vi "BoxExecute.vi"   [LabVIEW 2023]
uses:
  <vilib>/Rock Robotics/Network Tables/NT Write Number.vi
  <vilib>/Rock Robotics/Network Tables/NT Read Number.vi
  <vilib>/Rock Robotics/WPI/ThirdParty/JAS_Junk/TrajLib/Trajectory_Library.lvlib
  <vilib>/Rock Robotics/Network Tables/NT Write Boolean.vi
panel:
  # "Click here to set max"
  # "Click here to set min"
types:
  T1 = typedef "WPI_MotorControlDeviceRef.ctl" = cluster{"DeviceStatus":errorcluster, "Type":T2, "PWM":cluster{"PWM Channel":T3, "DeadBand":T4}, "CAN":cluster{"Device Number":u8, "SetOutput VI Ref":variant, "GetOutput VI Ref":variant, "Enable VI Ref":variant, "Disable VI Ref":variant, "Data":variant}, "Invert":bool, "DIO PWM":cluster{"PWM \"Enable\" Channel":T3, "DIOChannel":T5, "PWM Rate":dbl}}
  T2 = typedef "WPI_MotorControlType.ctl" = enum16{"PWM", "CAN", "DIO PWM"}
  T3 = typedef "FPGA_DIOPWMChannel.ctl" = enum8{"PWM 0", "PWM 1", "PWM 2", "PWM 3", "PWM 4", "PWM 5", "PWM 6", "PWM 7", "PWM 8", "PWM 9", "PWM MXP 0", "PWM MXP 1", "PWM MXP 2", "PWM MXP 3", "PWM MXP 4", "PWM MXP 5", "PWM MXP 6", "PWM MXP 7", "PWM MXP 8", "PWM MXP 9", "Invalid"}
  T4 = typedef "WPI_PWMDeadband.ctl" = cluster{"Name":string, "maxPositivePwm":i32, "minPositivePwm":i32, "centerPwm":i32, "maxNegativePwm":i32, "minNegativePwm":i32, "angularRange":u16}
  T5 = typedef "FPGA_DIOChannel.ctl" = enum8{"DIO 0", "DIO 1", "DIO 2", "DIO 3", "DIO 4", "DIO 5", "DIO 6", "DIO 7", "DIO 8", "DIO 9", "DIO MXP 0", "DIO MXP 1", "DIO MXP 2", "DIO MXP 3", "DIO MXP 4", "DIO MXP 5", "DIO MXP 6", "DIO MXP 7", "DIO MXP 8", "DIO MXP 9", "DIO MXP 10", "DIO MXP 11", "DIO MXP 12", "DIO MXP 13", "DIO MXP 14", "DIO MXP 15", "SPI Port CS1", "SPI Port CS2", "SPI Port CS3", "SPI Port MISO", "SPI Port MOSI", "Invalid"}
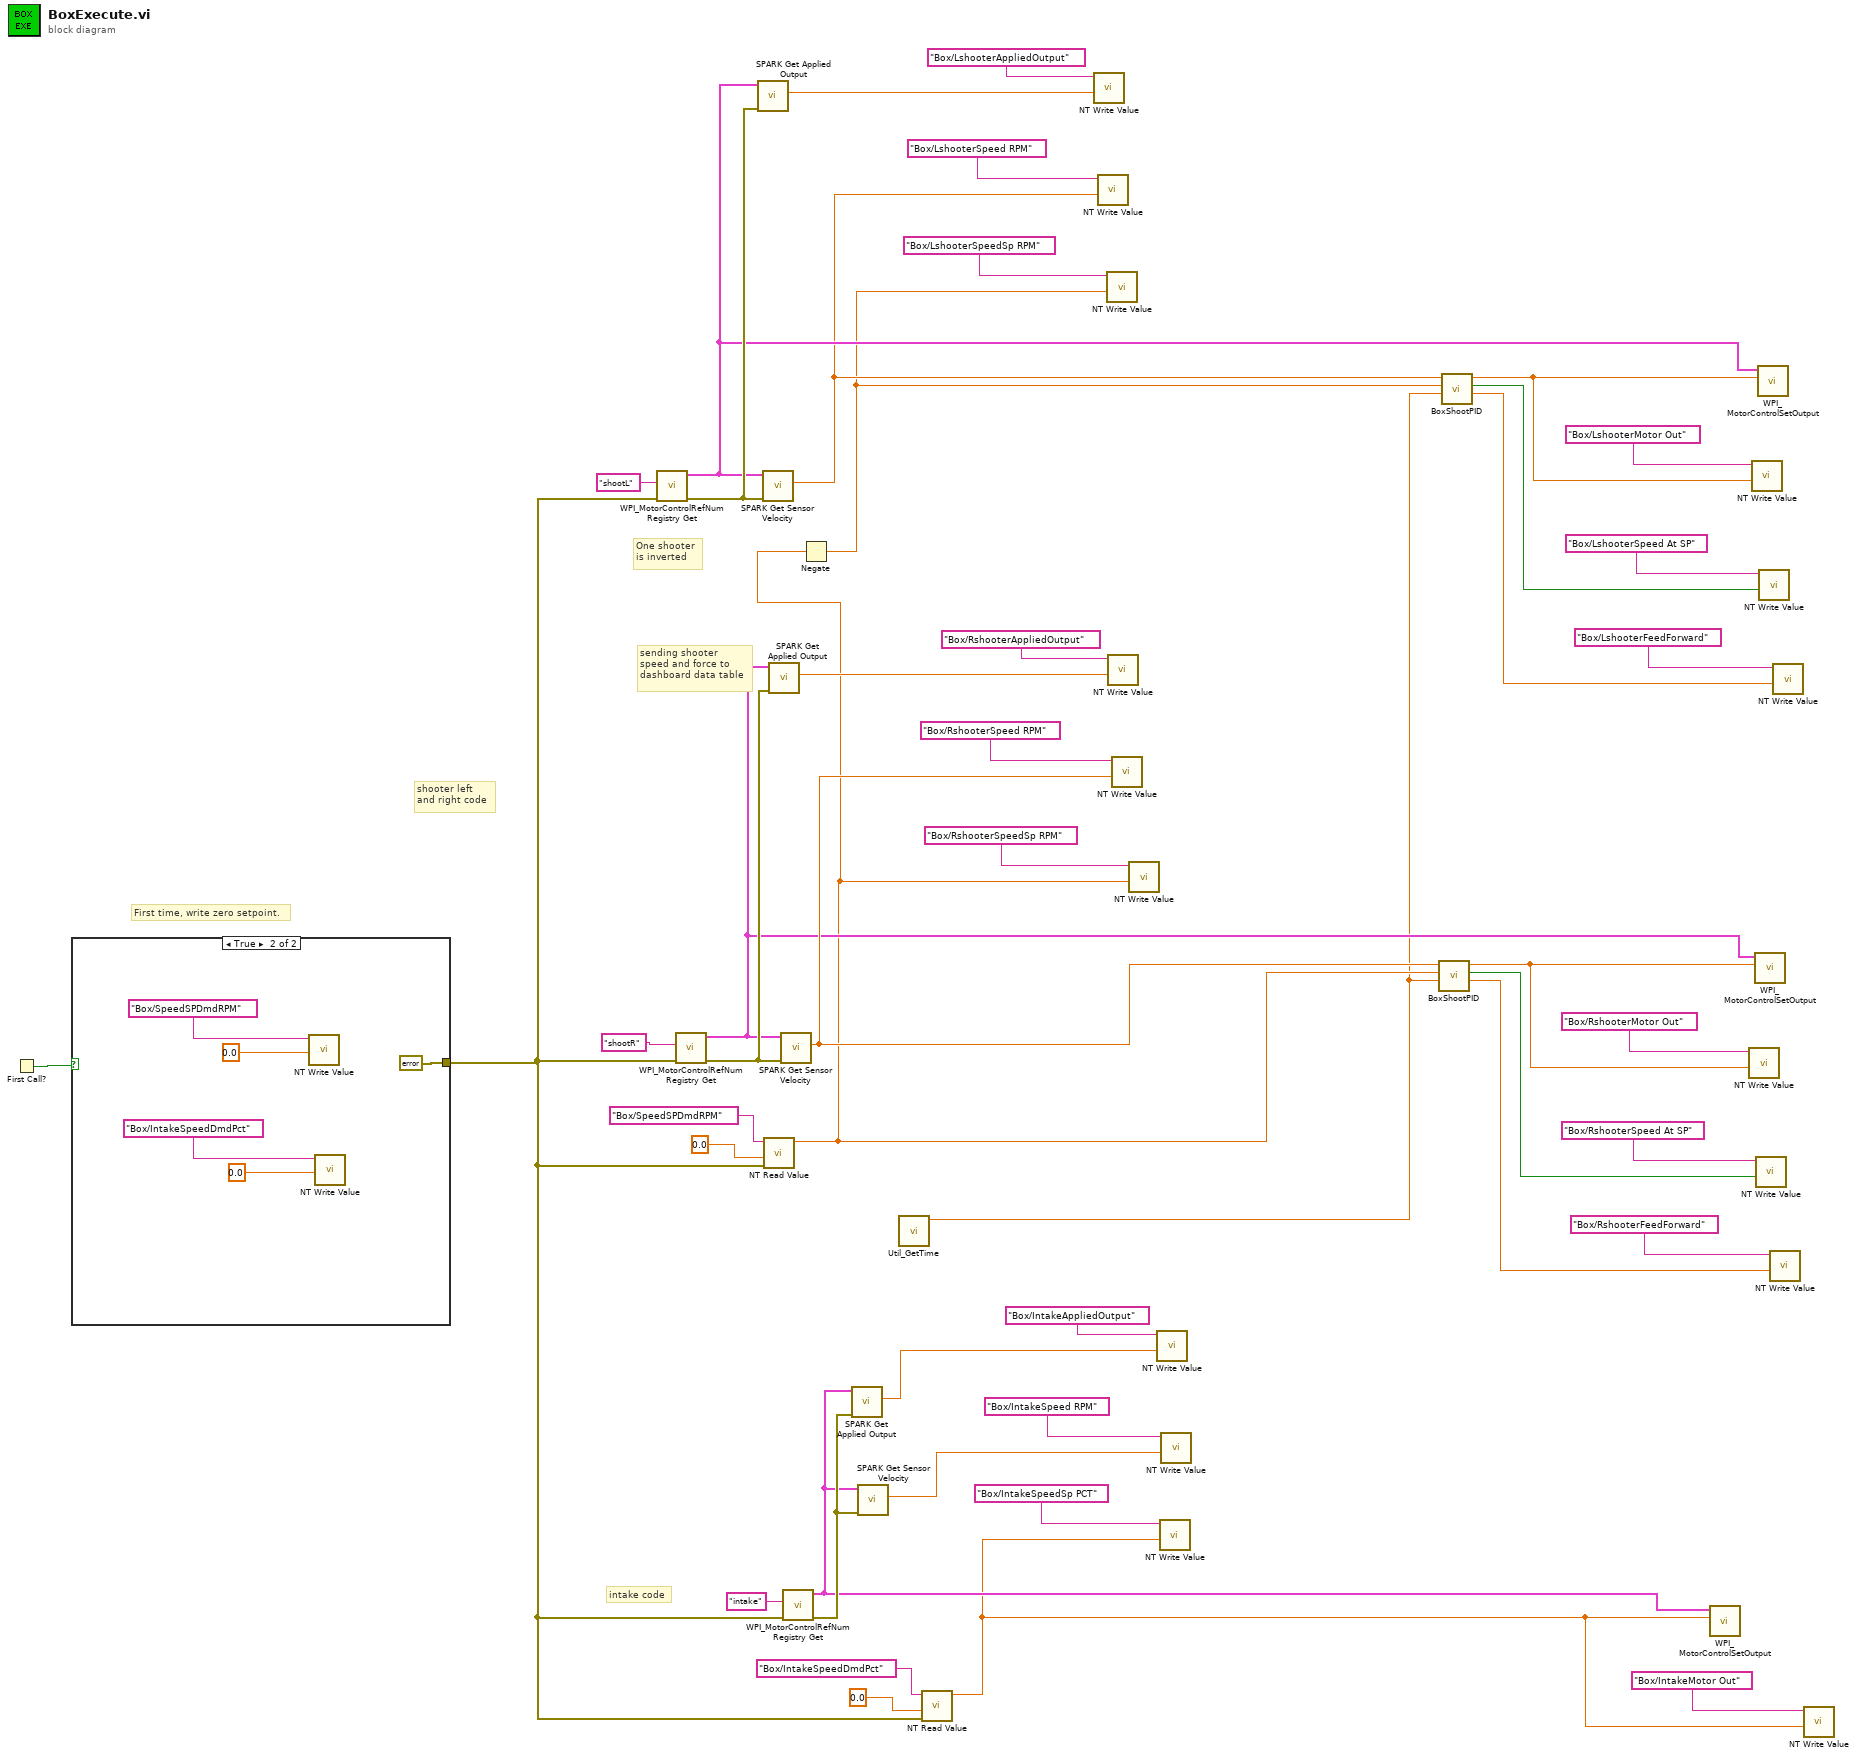
[diagram p0: block diagram]
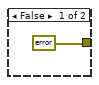
[diagram p2: hidden frame]
diagram:
  # "One shooter\nis inverted"
  # "First time, write zero setpoint."
  # "sending shooter \nspeed and force to\ndashboard data table"
  # "shooter left \nand right code"
  # "intake code"
  n1 = First Call?() -> (First Call?: T/F=w34:bool)
  n2 = case shown="True" w34 {
    tunnel: [errorcluster {"status"=FALSE, "code"=0, "source"=""} ("error in (no error)") errorcluster {"status"=FALSE, "code"=0, "source"=""} ("error in (no error)")] -> w5
    frame False {
    }
    frame True {
      n3 = call-poly <vilib>:"NT Write Value.vi"("value"=0.0, "name"="Box/SpeedSPDmdRPM") -> ()  [unwired: 9 in, 1 out]
      n4 = call-poly <vilib>:"NT Write Value.vi"("value"=0.0, "name"="Box/IntakeSpeedDmdPct") -> ()  [unwired: 9 in, 1 out]
    }
  }
  n5 = call <vilib>:"WPI_MotorControlRefNum Registry Get.vi"("error in (no error)"=w5, "refnum name"="shootL") -> ("error out"=w45:errorcluster, "MotorControlDevRef"=w16:T1)  [unwired: 8 in]
  n6 = call <vilib>:"WPI_MotorControlRefNum Registry Get.vi"("error in (no error)"=w5, "refnum name"="shootR") -> ("error out"=w43:errorcluster, "MotorControlDevRef"=w31:T1)  [unwired: 8 in]
  n7 = call <vilib>:"SPARK Get Applied Output.vi"("error in (no error)"=w45, "MotorControlDevRef in"=w16) -> ("Applied Output"=w40:dbl)  [unwired: 6 in, 3 out]
  n8 = call <vilib>:"SPARK Get Sensor Velocity.vi"("error in (no error)"=w45, "MotorControlDevRef in"=w16) -> ("Sensor Velocity"=w15:dbl)  [unwired: 6 in, 3 out]
  n9 = call-poly <vilib>:"NT Read Value.vi"("error in"=w5, "default value"=0.0, "name"="Box/SpeedSPDmdRPM") -> ("value"=w23:dbl)  [unwired: 6 in, 2 out]
  n10 = call <vilib>:"SPARK Get Applied Output.vi"("error in (no error)"=w43, "MotorControlDevRef in"=w31) -> ("Applied Output"=w37:dbl)  [unwired: 6 in, 3 out]
  n11 = call <vilib>:"SPARK Get Sensor Velocity.vi"("error in (no error)"=w43, "MotorControlDevRef in"=w31) -> ("Sensor Velocity"=w32:dbl)  [unwired: 6 in, 3 out]
  n12 = call <vilib>:"WPI_MotorControlRefNum Registry Get.vi"("error in (no error)"=w5, "refnum name"="intake") -> ("error out"=w10:errorcluster, "MotorControlDevRef"=w3:T1)  [unwired: 8 in]
  n13 = Negate(x=w23) -> (-x=w14:dbl)
  n14 = call <vilib>:"SPARK Get Applied Output.vi"("error in (no error)"=w10, "MotorControlDevRef in"=w3) -> ("Applied Output"=w9:dbl)  [unwired: 6 in, 3 out]
  n15 = call <vilib>:"SPARK Get Sensor Velocity.vi"("error in (no error)"=w10, "MotorControlDevRef in"=w3) -> ("Sensor Velocity"=w8:dbl)  [unwired: 6 in, 3 out]
  n16 = call <vilib>:"Util_GetTime.vi"() -> ("FPGA_Time_Seconds"=w13:dbl)  [unwired: 9 in, 2 out]
  n17 = call-poly <vilib>:"NT Read Value.vi"("error in"=w5, "default value"=0.0, "name"="Box/IntakeSpeedDmdPct") -> ("value"=w1:dbl)  [unwired: 6 in, 2 out]
  n18 = call-poly <vilib>:"NT Write Value.vi"("value"=w40, "name"="Box/LshooterAppliedOutput") -> ()  [unwired: 9 in, 1 out]
  n19 = call-poly <vilib>:"NT Write Value.vi"("value"=w15, "name"="Box/LshooterSpeed RPM") -> ()  [unwired: 9 in, 1 out]
  n20 = call-poly <vilib>:"NT Write Value.vi"("value"=w14, "name"="Box/LshooterSpeedSp RPM") -> ()  [unwired: 9 in, 1 out]
  n21 = call-poly <vilib>:"NT Write Value.vi"("value"=w37, "name"="Box/RshooterAppliedOutput") -> ()  [unwired: 9 in, 1 out]
  n22 = call-poly <vilib>:"NT Write Value.vi"("value"=w32, "name"="Box/RshooterSpeed RPM") -> ()  [unwired: 9 in, 1 out]
  n23 = call-poly <vilib>:"NT Write Value.vi"("value"=w23, "name"="Box/RshooterSpeedSp RPM") -> ()  [unwired: 9 in, 1 out]
  n24 = call-poly <vilib>:"NT Write Value.vi"("value"=w9, "name"="Box/IntakeAppliedOutput") -> ()  [unwired: 9 in, 1 out]
  n25 = call-poly <vilib>:"NT Write Value.vi"("value"=w1, "name"="Box/IntakeSpeedSp PCT") -> ()  [unwired: 9 in, 1 out]
  n26 = call-poly <vilib>:"NT Write Value.vi"("value"=w8, "name"="Box/IntakeSpeed RPM") -> ()  [unwired: 9 in, 1 out]
  n27 = call "BoxShootPID.vi"("FPGA_Time_Seconds"=w13, "Setpoint"=w23, "Sensor Velocity"=w32) -> ("FeedForward"=w25:dbl, "AtSetpoint"=w28:bool, "CO-ControlOutput"=w26:dbl)  [unwired: 6 in]
  n28 = call "BoxShootPID.vi"("FPGA_Time_Seconds"=w13, "Setpoint"=w14, "Sensor Velocity"=w15) -> ("FeedForward"=w17:dbl, "AtSetpoint"=w20:bool, "CO-ControlOutput"=w18:dbl)  [unwired: 6 in]
  n29 = call <vilib>:"WPI_MotorControlSetOutput.vi"("Output"=w1, "MotorControlDevRef"=w3) -> ()  [unwired: 7 in, 3 out]
  n30 = call-poly <vilib>:"NT Write Value.vi"("value"=w26, "name"="Box/RshooterMotor Out") -> ()  [unwired: 9 in, 1 out]
  n31 = call-poly <vilib>:"NT Write Value.vi"("value"=w18, "name"="Box/LshooterMotor Out") -> ()  [unwired: 9 in, 1 out]
  n32 = call <vilib>:"WPI_MotorControlSetOutput.vi"("Output"=w26, "MotorControlDevRef"=w31) -> ()  [unwired: 7 in, 3 out]
  n33 = call-poly <vilib>:"NT Write Value.vi"("value"=w28, "name"="Box/RshooterSpeed At SP") -> ()  [unwired: 9 in, 1 out]
  n34 = call <vilib>:"WPI_MotorControlSetOutput.vi"("Output"=w18, "MotorControlDevRef"=w16) -> ()  [unwired: 7 in, 3 out]
  n35 = call-poly <vilib>:"NT Write Value.vi"("value"=w20, "name"="Box/LshooterSpeed At SP") -> ()  [unwired: 9 in, 1 out]
  n36 = call-poly <vilib>:"NT Write Value.vi"("value"=w25, "name"="Box/RshooterFeedForward") -> ()  [unwired: 9 in, 1 out]
  n37 = call-poly <vilib>:"NT Write Value.vi"("value"=w17, "name"="Box/LshooterFeedForward") -> ()  [unwired: 9 in, 1 out]
  n38 = call-poly <vilib>:"NT Write Value.vi"("value"=w1, "name"="Box/IntakeMotor Out") -> ()  [unwired: 9 in, 1 out]
